vi "sort_scan_settings.vi"(7 "Scan settings array":T1[](array[typedef]) {"J-t settling delay (s)" min=10.0; "J-t illumination" items=["Light only", "Dark only", "Light then dark", "Dark then light"]; "Measurement speed" items=["Fast", "Normal", "High accuracy"]; "Illumination" items=["Light only", "Dark only", "Light then dark", "Dark then light"]; "Only repeat for best pixel" items=["only for best pixel", "for best 2 pixels", "for best 3 pixels", "for best 4 pixels", "for best 5 pixels", "for best 6 pixels", "for best 7 pixels", "for all pixels"]; "No. of repeat scans" min=1.0 step=1.0; "Max power best pixel only" items=["only the best pixel", "the best 2 pixels", "the best 3 pixels", "the best 4 pixels", "the best 5 pixels", "the best 6 pixels", "the best 7 pixels", "all pixels"]; "J-t best pixel only" items=["only the best pixel", "the best 2 pixels", "the best 3 pixels", "the best 4 pixels", "the best 5 pixels", "the best 6 pixels", "the best 7 pixels", "all pixels"]; "J-t measurement speed" items=["Fast", "Normal", "High Accuracy"]; "Stabilisation mode" items=["V", "I"]; "Measurement delay (ms)" min=10.0}, 10 "Setting name array":string[](array[string])) -> (0 "Sorted settings array":T1[](array[typedef]) {"J-t settling delay (s)" min=10.0; "J-t illumination" items=["Light only", "Dark only", "Light then dark", "Dark then light"]; "Measurement speed" items=["Fast", "Normal", "High accuracy"]; "Illumination" items=["Light only", "Dark only", "Light then dark", "Dark then light"]; "Only repeat for best pixel" items=["only for best pixel", "for best 2 pixels", "for best 3 pixels", "for best 4 pixels", "for best 5 pixels", "for best 6 pixels", "for best 7 pixels", "for all pixels"]; "No. of repeat scans" min=1.0 step=1.0; "Max power best pixel only" items=["only the best pixel", "the best 2 pixels", "the best 3 pixels", "the best 4 pixels", "the best 5 pixels", "the best 6 pixels", "the best 7 pixels", "all pixels"]; "J-t best pixel only" items=["only the best pixel", "the best 2 pixels", "the best 3 pixels", "the best 4 pixels", "the best 5 pixels", "the best 6 pixels", "the best 7 pixels", "all pixels"]; "J-t measurement speed" items=["Fast", "Normal", "High Accuracy"]; "Stabilisation mode" items=["V", "I"]; "Measurement delay (ms)" min=10.0}, 3 "Sorted name array":string[](array[string]))   [LabVIEW 2016]
uses:
  TypeDefs/scan_settings.ctl
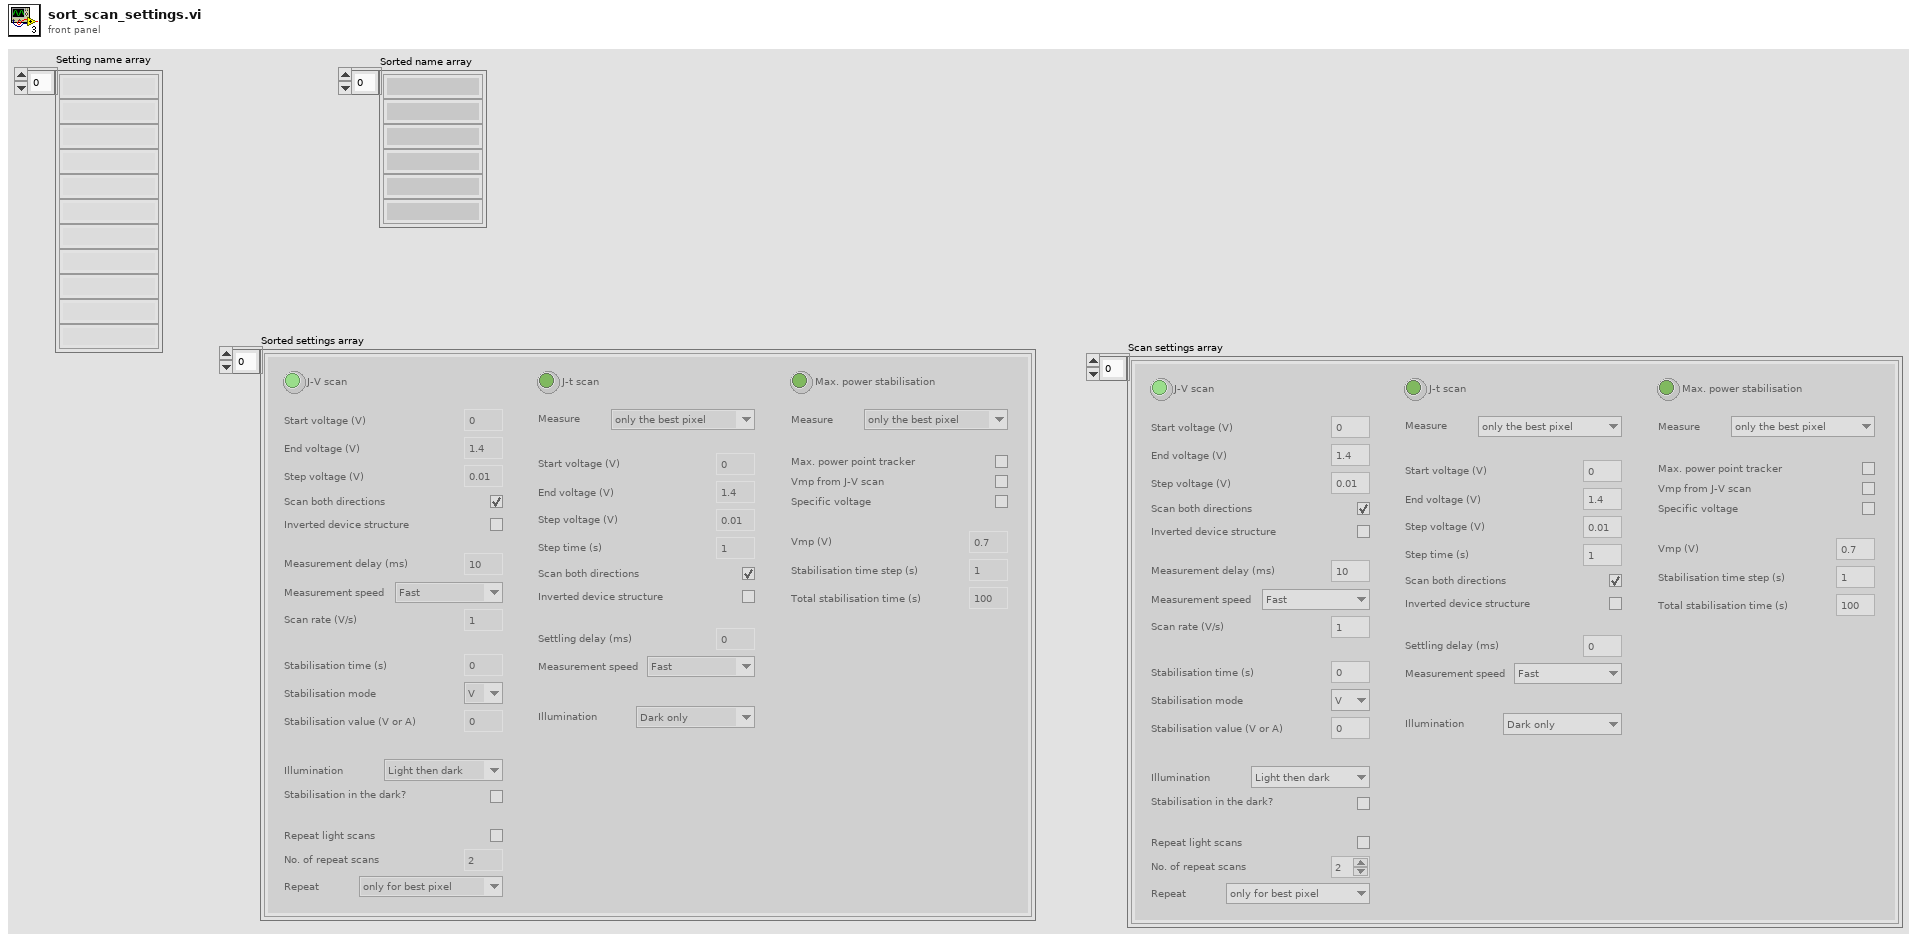
[diagram p1: front panel]
types:
  T1 = typedef "scan_settings.ctl" = cluster{"J-V scan":bool, "Start voltage (V)":dbl, "End voltage (V)":dbl, "Step voltage (V)":dbl, "Scan both directions":bool, "Inverted device structure":bool, "Measurement delay (ms)":dbl, "Measurement speed":u8, "Scan rate (V/s)":dbl, "Stabilisation time (s)":dbl, "Stabilisation mode":u16, "Stabilisation value (V or A) ":dbl, "Illumination":u16, "Stabilisation in the dark?":bool, "Repeat light scans":bool, "No. of repeat scans":dbl, "Only repeat for best pixel":u16, "J-t scan":bool, "J-t best pixel only":u16, "J-t start voltage (V)":dbl, "J-t end voltage (V)":dbl, "J-t step voltage (V)":dbl, "Step time (s)":dbl, "J-t scan both directions":bool, "J-t inverted device structure":bool, "J-t settling delay (s)":dbl, "J-t measurement speed":u16, "J-t illumination":u16, "Max. power stabilisation":bool, "Max power best pixel only":u16, "Max. power point tracker":bool, "Vmp from J-V scan":bool, "Max P stab. Specific voltage":bool, "Vmp (V)":dbl, "Stabilisation time step (s)":dbl, "Total stabilisation time (s)":dbl}
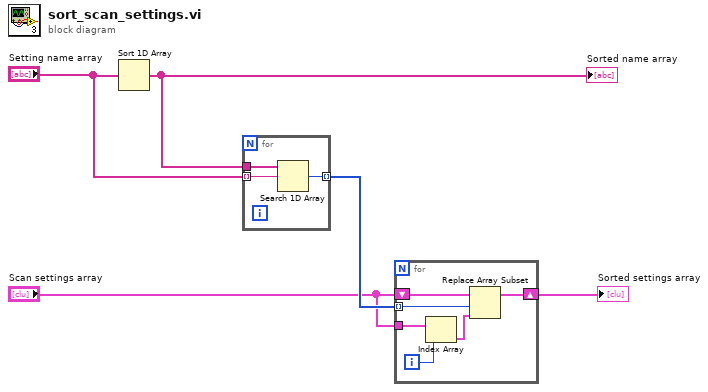
[diagram p0: block diagram]
diagram:
  n1 = Sort 1D Array(array="Setting name array") -> (sorted array=w5:string[])
  "Sorted name array" <- w5
  n2 = for {
    tunnel: w5 -> [w8]
    tunnel: "Setting name array" -> [w7] mode=indexing
    tunnel: [w6] -> w3 mode=indexing
    n3 = Search 1D Array(1D array=w8, element=w7) -> (index of element=w6:i32)  [unwired: 1 in]
  }
  n4 = for {
    shift-right: [w13] -> w2
    shift-left: "Scan settings array" -> [w14]
    tunnel: "Scan settings array" -> [w12]
    tunnel: w3 -> [w10] mode=indexing
    i -> [w9]
    n5 = Index Array(array=w12, index=w9) -> (element=w11:T1)
    n6 = Replace Array Subset(array=w14, new element=w11, index=w10) -> (w13:T1[])
  }
  "Sorted settings array" <- w2
